vi "Search Current.vi"(5 "BoardHandle in":T1, 11 "error in (no error)":errorcluster, 12 "Stop Program":bool) -> (1 "Actual Voltage Level (V)":dbl format="%#_13g", 2 "Power Supply Trip":bool, 3 "Actual Current Limit (nA)":dbl format="%#_13g", 10 "Measured Total Currents":dbl[](array[numeric]), 14 "BoardHandle out 2":T1, 15 "error out":errorcluster)   [LabVIEW 2020]
uses:
  Program Files/National Instruments/LabVIEW 2018/instr.lib/CAEN PSM/CAEN PSM.lvlib
panel:
  # "INPUTS"
  # "OUTPUTS"
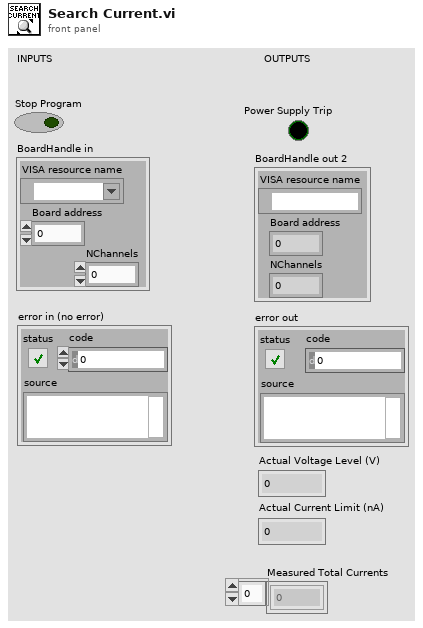
[diagram p1: front panel]
types:
  T1 = cluster{"VISA resource name":refnum<visa-resource-name>, "Board address":u8, "NChannels":u8}
  T2 = typedef "CAEN PSM.lvlib/BoardHandle.ctl" = cluster{"VISA resource name":refnum<visa-resource-name>, "Board address":u8, "NChannels":u8}
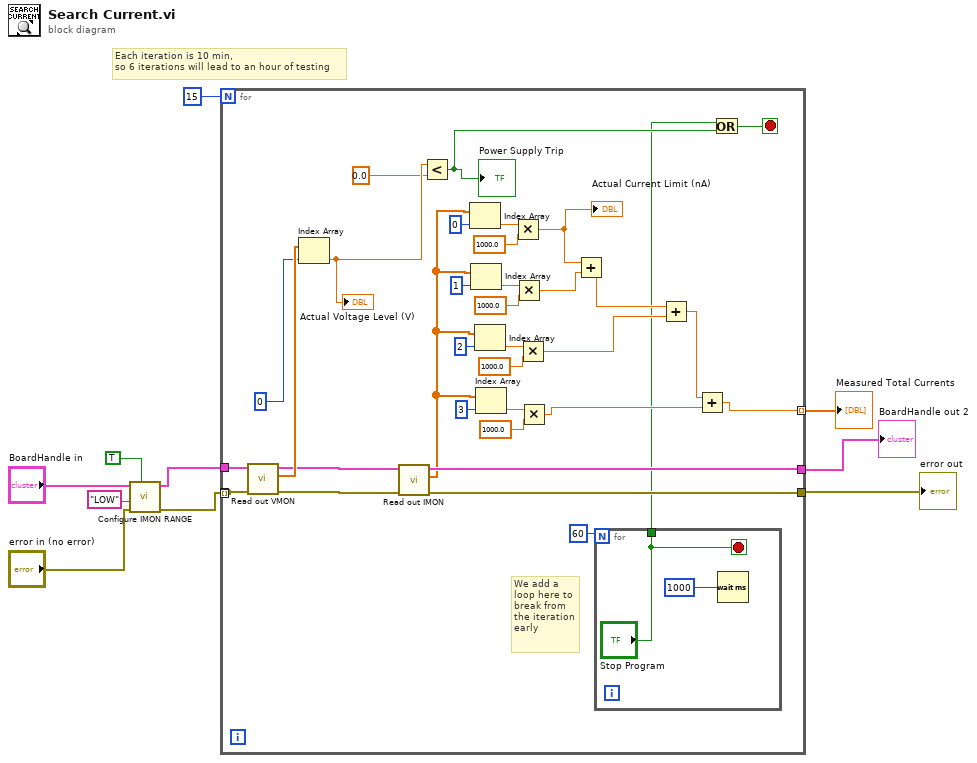
[diagram p0: block diagram]
diagram:
  # "Each iteration is 10 min,\nso 6 iterations will lead to an hour of testing"
  n1 = call "Configure IMON RANGE.vi"("All Channels (F)"=TRUE, "error in (no error)"="error in (no error)", "IMon range (LOW)"="LOW", "BoardHandle"="BoardHandle in") -> ("error out"=w4:errorcluster, "BoardHandle out"=w5:T2)  [unwired: 6 in]
  n2 = for {
    N: 15 ("N") -> [_]
    tunnel: w4 -> [w31]
    tunnel: [w41] -> w8
    tunnel: [w40] -> w9
    tunnel: [w18] -> w10 mode=indexing
    tunnel: w5 -> [w32]
    tunnel: [w31] -> _ mode=indexing
    stop <- w35 stop-if-true
    # "We add a \nloop here to\nbreak from \nthe iteration\nearly"
    n3 = call "Read out VMON.vi"("error in (no error)"=w31, "BoardHandle"=w32) -> ("error out"=w42:errorcluster, "VMon values (V)"=w44:dbl[], "BoardHandle out"=w43:T2)  [unwired: 7 in]
    n4 = Index Array(array=w44, index=0) -> (element=w37:dbl)
    "Actual Voltage Level (V)" <- w37
    n5 = call "Read out IMON.vi"("error in (no error)"=w42, "BoardHandle"=w43) -> ("error out"=w40:errorcluster, "IMon values (uA)"=w19:dbl[], "BoardHandle out"=w41:T2)  [unwired: 6 in, 1 out]
    n6 = Less?(x=w37, y=0.0) -> (x < y?=w34:bool)
    "Power Supply Trip" <- w34
    n7 = Index Array(array=w19, index=0) -> (element=w39:dbl)
    n8 = Index Array(array=w19, index=1) -> (element=w28:dbl)
    n9 = Index Array(array=w19, index=2) -> (element=w25:dbl)
    n10 = Index Array(array=w19, index=3) -> (element=w22:dbl)
    n11 = Multiply(x=w39, y=1000.0) -> (x*y=w14:dbl)
    "Actual Current Limit (nA)" <- w14
    n12 = Multiply(x=w28, y=1000.0) -> (x*y=w13:dbl)
    n13 = Multiply(x=w25, y=1000.0) -> (x*y=w12:dbl)
    n14 = Multiply(x=w22, y=1000.0) -> (x*y=w17:dbl)
    n15 = Add(x=w14, y=w13) -> (x+y=w15:dbl)
    n16 = for {
      N: 60 ("dt (s) in") -> [_]
      tunnel: ["Stop Program"] -> w11
      stop <- "Stop Program" stop-if-true
      n17 = Wait (ms)(milliseconds to wait=1000) -> ()  [unwired: 1 out]
    }
    n18 = Add(x=w15, y=w12) -> (x+y=w16:dbl)
    n19 = Add(x=w16, y=w17) -> (x+y=w18:dbl)
    n20 = Or(x=w11, y=w34) -> (x .or. y?=w35:bool)
  }
  "Measured Total Currents" <- w10
  "error out" <- w9
  "BoardHandle out 2" <- w8
